vi "Global State Variables.vi"() -> ()   [LabVIEW 2016]
panel:
  in  "DriveSpeedRange":enum16{"DriveSpeedHigh", "DriveSpeedLow"}(ring)
  in  "WinchState":enum16{"WinchOff", "WinchClimb", "WinchHold"}(ring)
  in  "Camera Selected":enum16{"Peg Camera", "Rope Camera"}(ring)
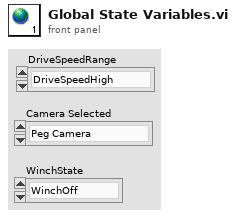
[diagram p1: front panel]
diagram:
